vi "VMI_clean_up_Camera.vi"(4 "Error In":errorcluster, 5 "Run Options":u16(ring)=1 items=["Collect Camera", "Test with Image"], 6 "Camera Session":T1) -> (0 "Error Out":errorcluster)   [LabVIEW 2019]
uses:
  <vilib>/userDefined/High Color/IMAQdx.ctl
  <vilib>/vision/driver/NI_Vision_Acquisition_Software.lvlib
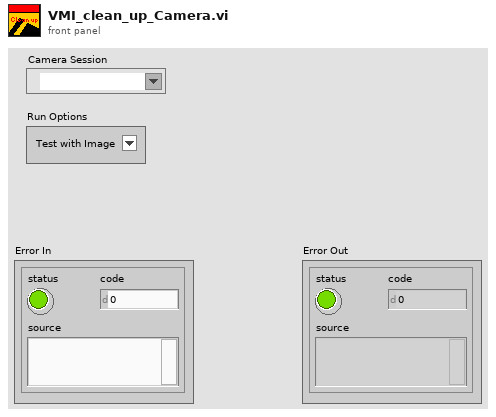
[diagram p1: front panel]
types:
  T1 = typedef "IMAQdx.ctl" = refnum<k21>
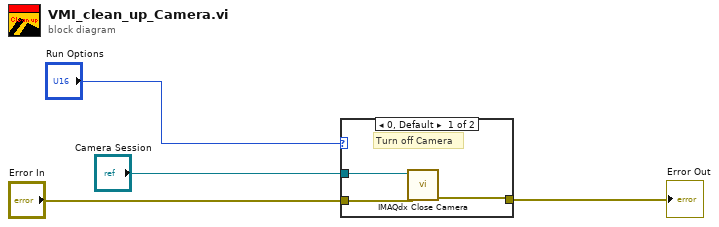
[diagram p0: block diagram]
diagram:
  n1 = case shown="0, Default" "Run Options" {
    tunnel: "Error In" -> [w6 w8]
    tunnel: "Camera Session" -> [w7 _]
    tunnel: [w5 w8] -> w1
    frame 0, Default {
      # "Turn off Camera"
      n2 = call <vilib>:"IMAQdx Close Camera.vi"("error in"=w6, "Session In"=w7) -> ("error out"=w5:errorcluster)  [unwired: 9 in]
    }
    frame 1 {
    }
  }
  "Error Out" <- w1
